vi "TestStep AllowAsynchronous.vi"(8 "error in (no error)":errorcluster, 11 "niDTS Test in":refnum<class "niDTS BT Rx Test.lvclass">) -> (0 "error out":errorcluster, 2 "AllowAsynchronous":bool=TRUE, 3 "niDTS Test out":refnum<class "niDTS BT Rx Test.lvclass">)   [LabVIEW 2015, in "niDTS BT.lvlib" / "niDTS BT Rx Test.lvclass"]
uses:
  niDTS BT Rx Test.lvclass
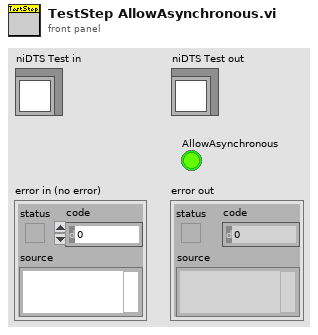
[diagram p1: front panel]
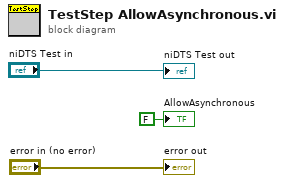
[diagram p0: block diagram]
diagram:
  "error out" <- "error in (no error)"
  "niDTS Test out" <- "niDTS Test in"
  "AllowAsynchronous" <- FALSE ("AllowAsynchronous")
